vi "Generate basic information.vi"(8 "error in":errorcluster caption="에러 입력(에러 없음)", 11 "RawDataSheet":path caption="템플릿(비어있음)") -> (0 "error out":errorcluster caption="에러 출력", 3 "참 버튼?":bool, 4 "파일이름":string)   [LabVIEW 2020]
uses:
  <vilib>/Utility/NIReport.llb/Report Type.ctl
  <vilib>/Utility/error.llb/DialogType.ctl
  <vilib>/Utility/NIReport.llb/NI_report.lvclass
  <vilib>/Utility/NIReport.llb/NI_ReportGenerationCore.lvlib
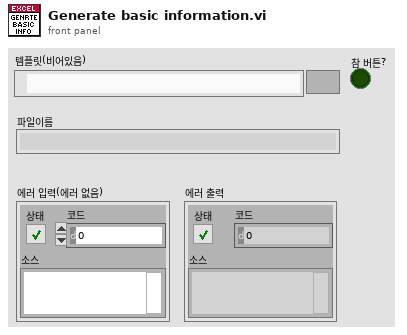
[diagram p1: front panel]
types:
  T1 = typedef "NI_ReportGenerationCore.lvlib/Report Type.ctl" = enum16{"HTML", "Word", "Excel"}
  T2 = enum16{"maximized", "minimized", "normal", "no change"}
  T3 = typedef "DialogType.ctl" = u16
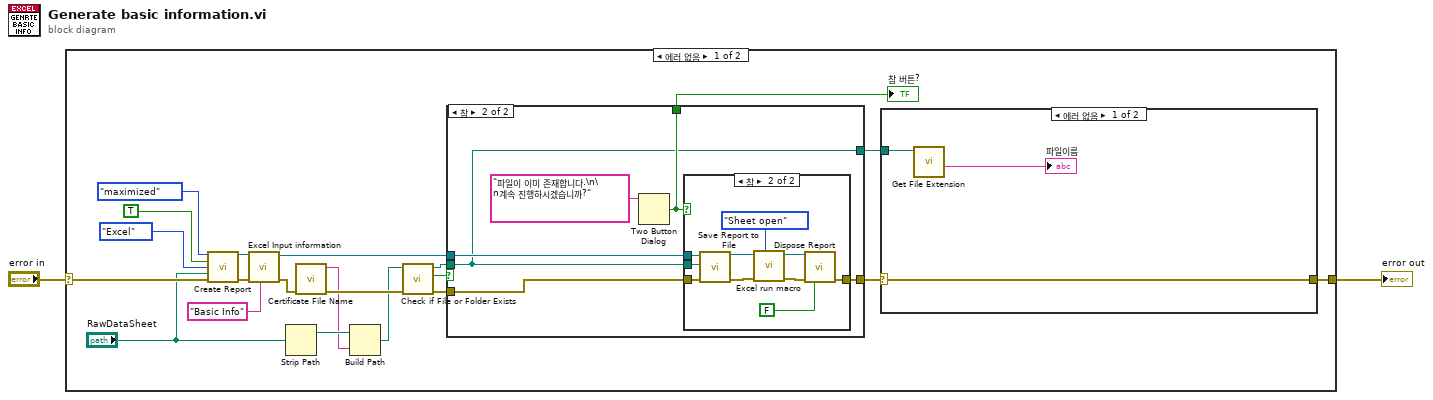
[diagram p0: block diagram]
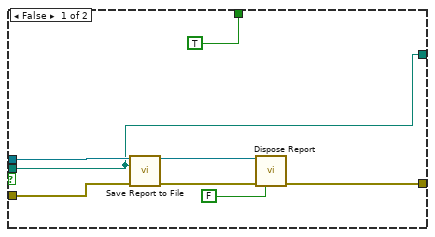
[diagram p2: hidden frame]
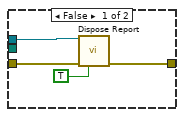
[diagram p3: hidden frame]
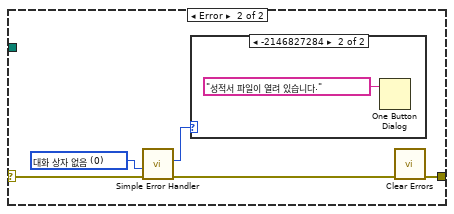
[diagram p4: hidden frame]
diagram:
  n1 = case shown="에러 없음" "error in" {
    selector: "error in" -> [w22 w61]
    tunnel: [w17 w61] -> w1
    frame No Error {
      n2 = call <vilib>:"Create Report.vi"("window state (normal)"=T2."maximized", "display alerts? (F)"=TRUE, "report type"=Report_Type."Excel", "template (empty)"="RawDataSheet", "error in (no error)"=w22) -> ("report out"=w20:refnum<class "NI_report.lvclass">, "error out"=w21:errorcluster)  [unwired: 9 in]
      n3 = call "Excel Input information.vi"("문자열"="Basic Info", "error in"=w21, "report in"=w20) -> ("error out"=w16:errorcluster, "report out"=w9:refnum<class "NI_report.lvclass">)  [unwired: 7 in]
      n4 = Strip Path(path="RawDataSheet") -> (stripped path=w15:path)  [unwired: 1 out]
      n5 = call "Certificate File Name.vi"("error in (no error)"=w16) -> ("error out"=w14:errorcluster, "성적서 파일명"=w8:string)  [unwired: 8 in, 1 out]
      n6 = Build Path(base path=w15, name or relative path=w8) -> (appended path=w13:path)
      n7 = call <vilib>:"Check if File or Folder Exists.vi"("error in (no error)"=w14, "path"=w13) -> ("error out"=w12:errorcluster, "file or folder exists?"=w11:bool, "dup path"=w10:path)  [unwired: 7 in]
      n8 = case shown="참" w11 {
        tunnel: w9 -> [w31 w35]
        tunnel: w12 -> [w30 w36]
        tunnel: w10 -> [w24 w32]
        tunnel: [w28 w34] -> w18
        tunnel: [TRUE ("T button?") w33] -> w6
        tunnel: [w24 w32] -> w3
        frame False {
          n9 = call-dynamic "Save Report to File.vi"("report in"=w31, "report file path"=w24, "error in (no error)"=w30) -> ("report out"=w26:refnum<class "NI_report.lvclass">, "error out"=w29:errorcluster)  [unwired: 11 in]
          n10 = call-dynamic "Dispose Report.vi"("report in"=w26, "error in (no error)"=w29, "close report? (T)"=FALSE) -> ("error out"=w28:errorcluster)  [unwired: 12 in]
        }
        frame True {
          n11 = Two Button Dialog(message="파일이 이미 존재합니다.\n\n계속 진행하시겠습니까?" ("메시지")) -> (T button?=w33:bool)  [unwired: 2 in]
          n12 = case shown="참" w33 {
            tunnel: w36 -> [w41 w51]
            tunnel: w35 -> [w39 w50]
            tunnel: [w40 w48] -> w34
            tunnel: w32 -> [_ w47]
            frame False {
              n13 = call-dynamic "Dispose Report.vi"("report in"=w39, "error in (no error)"=w41, "close report? (T)"=TRUE) -> ("error out"=w40:errorcluster)  [unwired: 12 in]
            }
            frame True {
              n14 = call-dynamic "Save Report to File.vi"("report in"=w50, "report file path"=w47, "error in (no error)"=w51) -> ("report out"=w45:refnum<class "NI_report.lvclass">, "error out"=w43:errorcluster)  [unwired: 11 in]
              n15 = call "Excel run macro.vi"("Comm"=enum16{"Protect", "Delete_Sheets", "Sheet open"}."Sheet open", "error in"=w43, "report in"=w45) -> ("error out"=w42:errorcluster, "report out"=w44:refnum<class "NI_report.lvclass">)  [unwired: 7 in]
              n16 = call-dynamic "Dispose Report.vi"("report in"=w44, "error in (no error)"=w42, "close report? (T)"=FALSE) -> ("error out"=w48:errorcluster)  [unwired: 12 in]
            }
          }
        }
      }
      "참 버튼?" <- w6
      n17 = case shown="에러 없음" w18 {
        selector: w18 -> [w54 w58]
        tunnel: [w54 w59] -> w17
        tunnel: w3 -> [w53 _]
        frame No Error {
          n18 = call <vilib>:"Get File Extension.vi"("file"=w53) -> ("filename without extension"=→"파일이름":string)  [unwired: 6 in, 4 out]
        }
        frame Error {
          w55 = T3 0 items=["대화 상자 없음", "확인 메시지", "메시지 지속 또는 정지", "확인 메시지 + 경고", "지속/정지 + 경고"] ("type of dialog (OK msg:1)")
          n19 = call <vilib>:"Simple Error Handler.vi"("type of dialog (OK msg:1)"=w55, "error in (no error)"=w58) -> ("code out"=w56:i32, "error out"=w57:errorcluster)  [unwired: 3 in, 3 out]
          n20 = case shown="-2146827284" w56 {
            frame 0, Default {
            }
            frame -2146827284 {
              n21 = One Button Dialog(message="성적서 파일이 열려 있습니다." ("메시지")) -> ()  [unwired: 1 in, 1 out]
            }
          }
          n22 = call <vilib>:"Clear Errors.vi"("error in (no error)"=w57) -> ("error out"=w59:errorcluster)  [unwired: 5 in, 1 out]
        }
      }
    }
    frame Error {
    }
  }
  "error out" <- w1
